vi "Add Row to Listbox.vi"(6 "List size":i32=23, 8 "error in":errorcluster, 10 "Teszt cluster":T1, 11 "MulticolumnListbox in":refnum<vi>) -> (0 "error out":errorcluster)   [LabVIEW 2014]
uses:
  Teszt/Teszt.ctl
  Teszt/Command.ctl
  <vilib>/Utility/miscctls.llb/LVRowAndColumnTypeDef.ctl
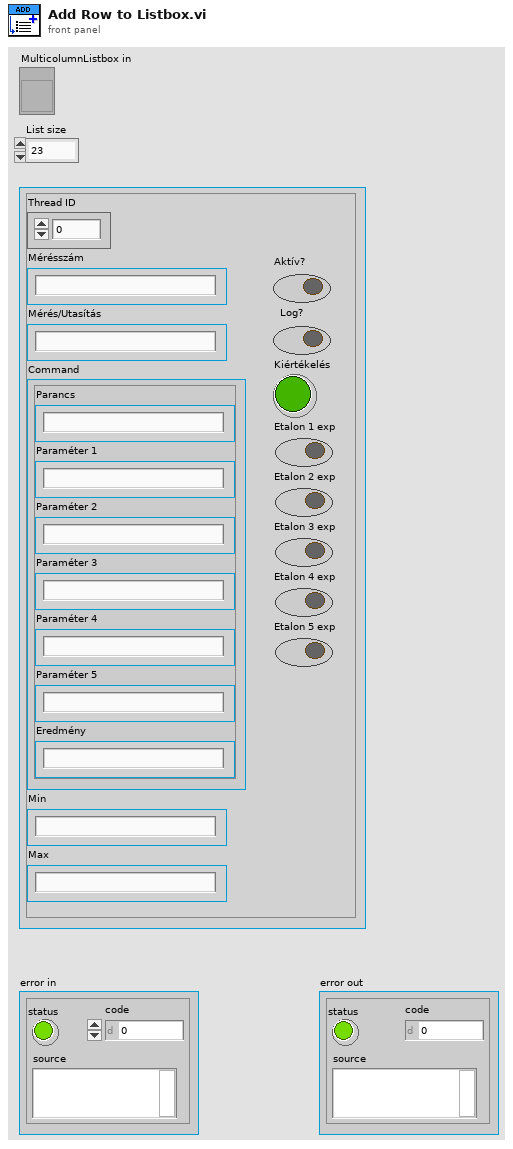
[diagram p1: front panel]
types:
  T1 = typedef "Teszt.ctl" = cluster{"Thread ID":dbl, "Mérésszám":string, "Mérés/Utasítás":string, "Command":T2, "Min":string, "Max":string, "Aktív?":bool, "Log?":bool, "Kiértékelés":bool, "Etalon 1 exp":bool, "Etalon 2 exp":bool, "Etalon 3 exp":bool, "Etalon 4 exp":bool, "Etalon 5 exp":bool}
  T2 = typedef "Command.ctl" = cluster{"Parancs":string, "Paraméter 1":string, "Paraméter 2":string, "Paraméter 3":string, "Paraméter 4":string, "Paraméter 5":string, "Eredmény":string}
  T3 = typedef "LVRowAndColumnTypeDef.ctl" = cluster{"Row":i32, "Column":i32}
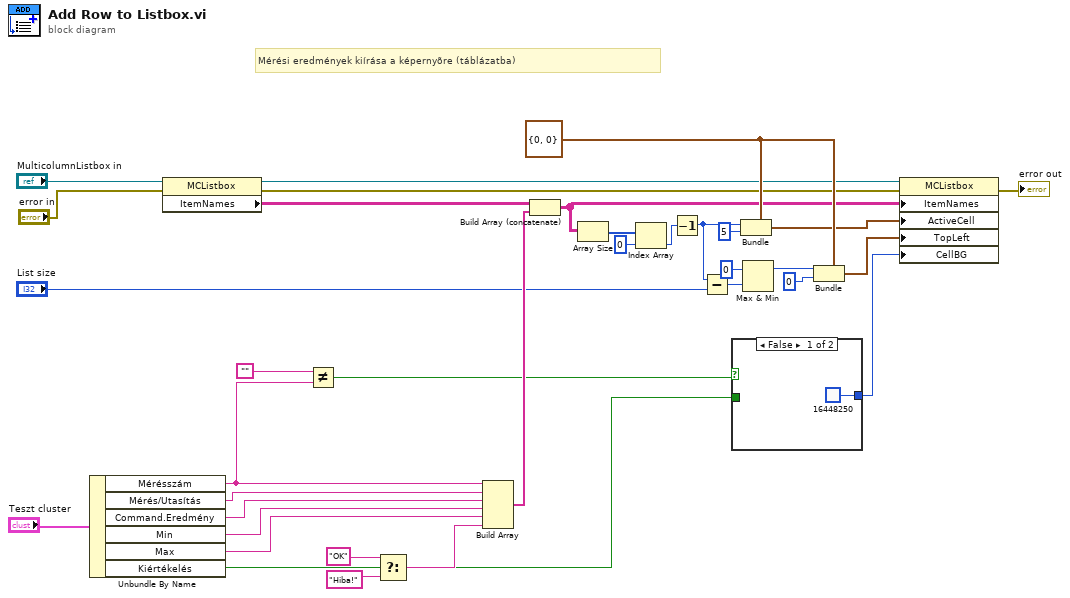
[diagram p0: block diagram]
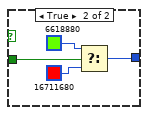
[diagram p2: hidden frame]
diagram:
  w13 = T3 {"Row"=0, "Column"=0} ("Active Cell:Active Cell")
  # "Mérési eredmények kiírása a képernyõre (táblázatba)"
  n1 = Unbundle By Name("Teszt cluster") -> ("Mérésszám"=w3:string, "Mérés/Utasítás"=w30:string, "Command.Eredmény"=w29:string, "Min"=w28:string, "Max"=w27:string, "Kiértékelés"=w26:bool)
  n2 = property class="MCListbox"(reference="MulticolumnListbox in", error in="error in") -> (reference out=w11:refnum<vi>, error out=w10:errorcluster, "ItemNames"=w8:string[][])
  n3 = Not Equal?(x="", y=w3) -> (x != y?=w1:bool)
  n4 = Select(t="OK", s=w26, f="Hiba!") -> (s? t:f=w34:string)
  n5 = Build Array(w3, w30, w29, w28, w27, w34) -> (w24:string[])
  n6 = Build Array (concatenate)(w8, w24) -> (w7:string[][])
  n7 = Array Size(array=w7) -> (size(s)=w21:i32[])
  n8 = Index Array(array=w21, index=0) -> (element=w23:i32)
  n9 = Decrement(x=w23) -> (x-1=w17:i32)
  n10 = Subtract(x=w17, y="List size") -> (x-y=w18:i32)
  n11 = case shown="False" w1 {
    tunnel: w26 -> [_ w39]
    tunnel: [u32 16448250 w36] -> w4
    frame False {
    }
    frame True {
      n12 = Select(t=u32 6618880, s=w39, f=u32 16711680) -> (s? t:f=w36:u32)
    }
  }
  n13 = Bundle(cluster=w13, "Row"=w17, "Column"=5) -> (w9:T3)
  n14 = Max & Min(x=0, y=w18) -> (max(x,y)=w15:i32)  [unwired: 1 out]
  n15 = Bundle(cluster=w13, "Row"=w15, "Column"=0) -> (w12:T3)
  n16 = property class="MCListbox"(reference=w11, error in=w10, "ItemNames"=w7, "ActiveCell"=w9, "TopLeft"=w12, "CellBG"=w4) -> (error out=→"error out":errorcluster)  [unwired: 1 out]
